vi "Get Error.vi"(0 "VISA resource name":refnum<visa-resource-name>, 11 "error in (no error)":errorcluster) -> (4 "VISA resource name out":refnum<visa-resource-name>, 15 "error out":errorcluster)   [LabVIEW 2023, in "ACM Visa Driver.lvlib"]
uses:
  ACM Visa Driver.lvlib
  <vilib>/Utility/error.llb/Trim Whitespace One-Sided.vi
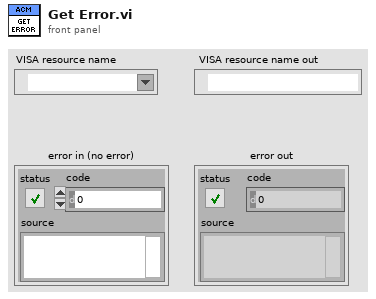
[diagram p1: front panel]
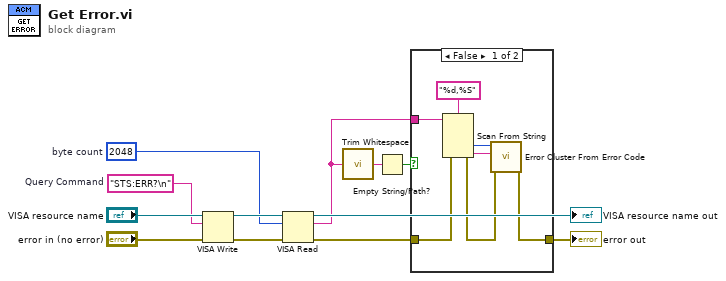
[diagram p0: block diagram]
diagram:
  w6 = u32 2048  # byte count
  w7 = "STS:ERR?\n"  # Query Command
  n1 = VISA Write(VISA resource name="VISA resource name", write buffer=w7, error in (no error)="error in (no error)") -> (VISA resource name out=w10:refnum<visa-resource-name>, error out=w11:errorcluster)  [unwired: 1 out]
  n2 = VISA Read(VISA resource name=w10, byte count=w6, error in (no error)=w11) -> (VISA resource name out=→"VISA resource name out":refnum<visa-resource-name>, read buffer=w3:string, error out=w4:errorcluster)  [unwired: 1 out]
  n3 = call <vilib>:"Trim Whitespace.vi"("string"=w3) -> ("trimmed string"=w2:string)  [unwired: 1 in]
  n4 = Empty String/Path?(string/path=w2) -> (empty?=w1:bool)
  n5 = case shown="False" w1 {
    tunnel: [w16 w20] -> w5
    tunnel: w4 -> [w15 w20]
    tunnel: w3 -> [w13 _]
    frame False {
      n6 = Scan From String(format string="%d,%S", input string=w13, error in=w15) -> (error out=w14:errorcluster, output 1=w18:i32, output 2=w17:string)  [unwired: 3 in, 2 out]
      n7 = call <vilib>:"Error Cluster From Error Code.vi"("error in (no error)"=w14, "error message (\"\")"=w17, "error code (0)"=w18) -> ("error out"=w16:errorcluster)  [unwired: 6 in]
    }
    frame True {
    }
  }
  "error out" <- w5
